vi "rmx13_rev2.vi"() -> ()   [LabVIEW 2012]
uses:
  <vilib>/Utility/inputDevices.llb/closeKeyboard.vi
  <vilib>/Utility/inputDevices.llb/keyboardAcquire.vi
panel:
  in  "Tab Control":enum32{"Front Panel"}(tab)
  out "excavator direction":string="a"
  out "bot direction":string="a"
  out "excavator state":string="a"
  out "hopper state":string="a"
  out "bytes written":i32
  out "tx'd string":string
  out "error out":errorcluster
  in  "Boolean 2":bool
  in  "Boolean":bool
  out "Total Elapsed Time  (HH:MM:SS)":dbl format="%<%H:%M:%S%2u>t"
  out "hup":bool
  out "hdown":bool
  out "xfwd":bool
  out "xback":bool
  out "xdown":bool
  out "xup":bool
  out "right":bool
  out "left":bool
  out "down":bool
  out "up":bool
  # "Excavator State"
  # "Elapsed Time"
  # "Error Control"
  # "Dump Position"
  # "Excavator Direction"
  # "Start/Stop"
  # "Bot Direction"
  # "Hopper State"
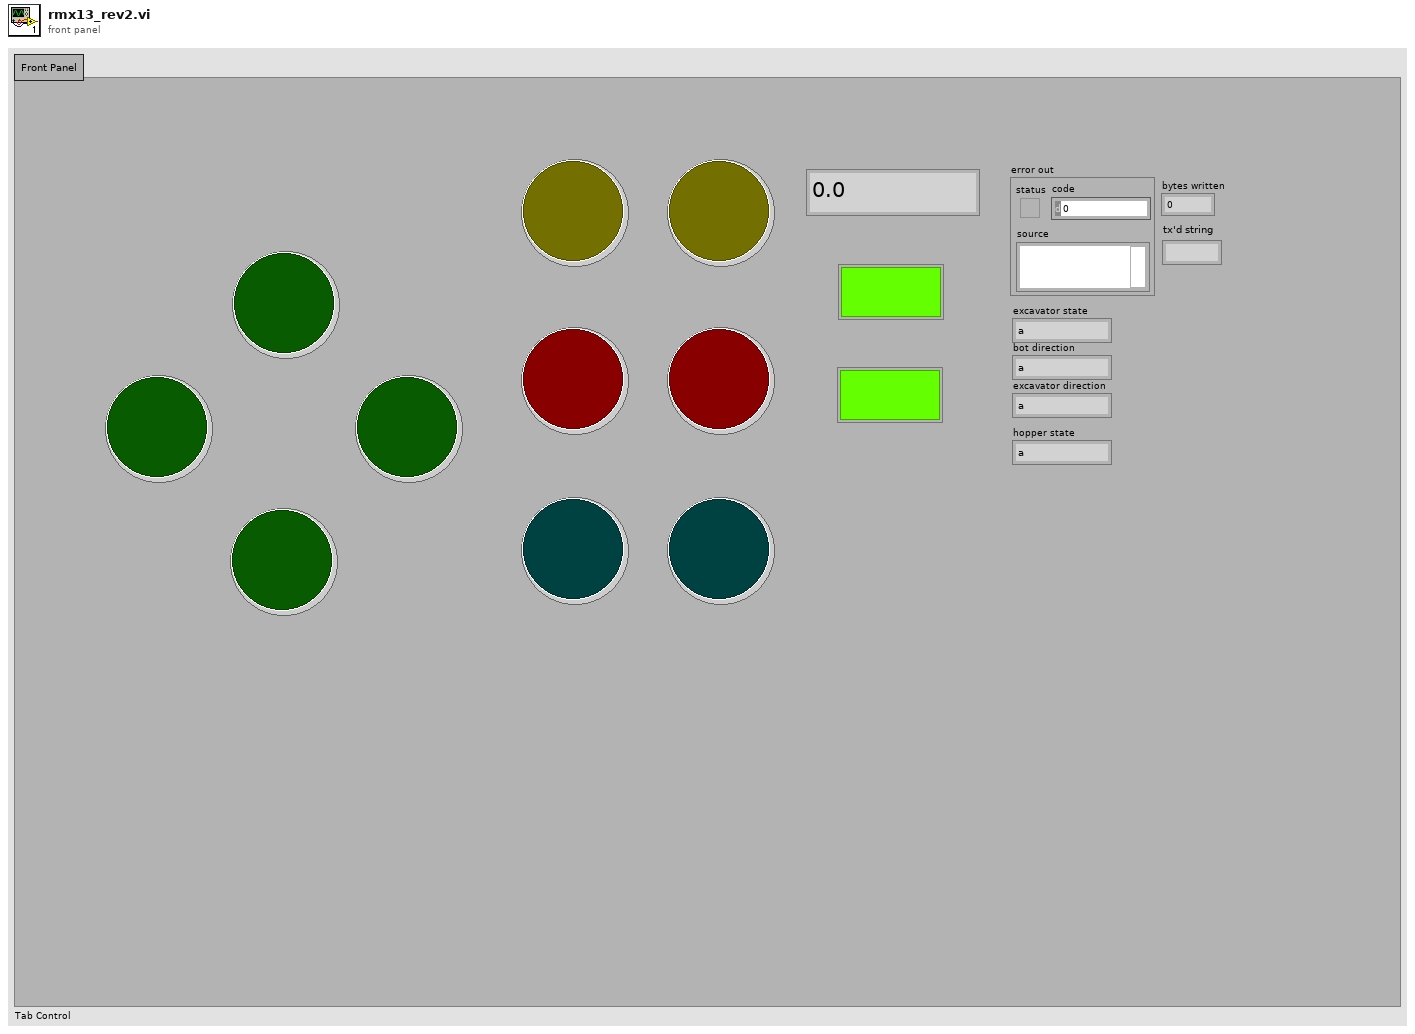
[diagram p1: front panel]
types:
  T1 = enum16{"0", "1", "2", "3", "4", "5", "6", "7", "8", "9", "A", "B", "C", "D", "E", "F", "G", "H", "I", "J", "K", "L", "M", "N", "O", "P", "Q", "R", "S", "T", "U", "V", "W", "X", "Y", "Z", "F1", "F2", "F3", "F4", "F5", "F6", "F7", "F8", "F9", "F10", "F11", "F12", "F13", "F14", "F15", "ADD", "BACK", "BACKSLASH", "CAPITAL", "COMMA", "DECIMAL", "DELETE", "DIVIDE", "DOWN", "END", "EQUALS", "ESCAPE", "GRAVE (`)", "HOME", "INSERT", "LBRACKET", "LCONTROL", "LEFT", "L ALT", "LSHIFT", "LWIN", "MINUS", "MULTIPLY", "NEXT", "NUMLOCK", "NUMPAD_0", "NUMPAD_1", "NUMPAD_2", "NUMPAD_3", "NUMPAD_4", "NUMPAD_5", "NUMPAD_6", "NUMPAD_7", "NUMPAD_8", "NUMPAD_9", "PAUSE", "PERIOD", "PRIOR (PG UP)", "RBRACKET", "RCONTROL", "RETURN", "RIGHT", "R ALT", "RSHIFT", "RWIN", "SCROLL", "SEMICOLON", "SLASH", "SPACE", "SUBTRACT", "TAB", "UP", "ENTER (num pad)", "' (quote)"}[]
  T2 = cluster{"up":bool, "down":bool, "left":bool, "right":bool, "xup":bool, "xdown":bool, "hup":bool, "hdown":bool, "xfwd":bool, "xback":bool}
  T3 = cluster{"bot_dir":string, "x-state":string, "h-state":string, "x-dir":string}
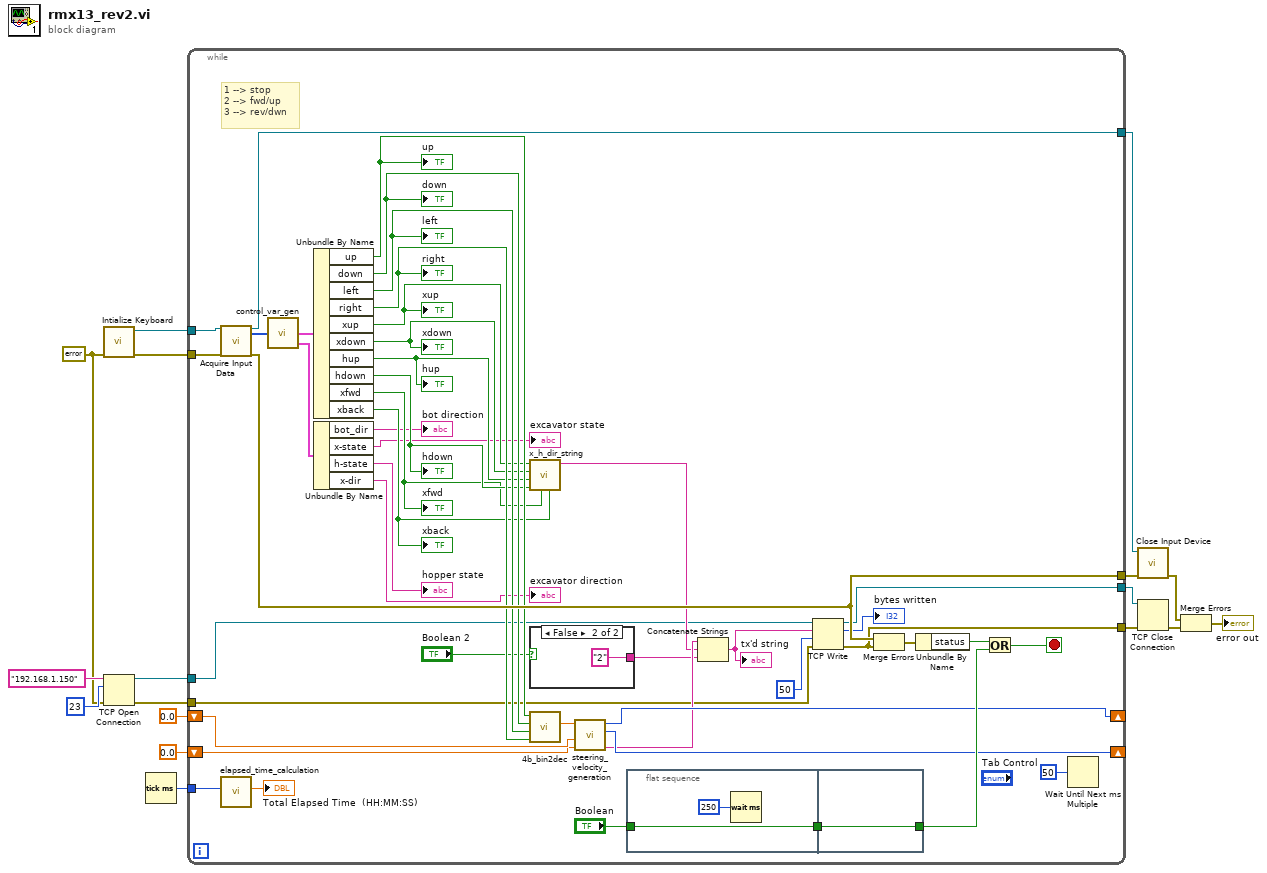
[diagram p0: block diagram]
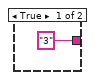
[diagram p2: hidden frame]
diagram:
  w3 = errorcluster {"status"=FALSE, "code"=0, "source"=""} ("error in")
  n1 = call <vilib>:"Intialize Keyboard.vi"("error in (no error)"=w3) -> ("error out"=w16:errorcluster, "device ID"=w17:refnum<k1>)  [unwired: 9 in]
  n2 = TCP Open Connection(address="192.168.1.150", remote port or service name=u16 23, error in (no error)=w3) -> (connection ID=w6:refnum<k5>, error out=w7:errorcluster)  [unwired: 2 in]
  n3 = Tick Count (ms)() -> (millisecond timer value=w13:u32)
  n4 = while {
    tunnel: w17 -> [w63]
    tunnel: w16 -> [w62]
    tunnel: [w59] -> w15
    tunnel: [w51] -> w14
    tunnel: w13 -> [w44]
    shift-right: [w46] -> _
    shift-left: 0.0 -> [w48]
    shift-right: [w45] -> _
    shift-left: 0.0 -> [w47]
    tunnel: w7 -> [w30]
    tunnel: w6 -> [w29]
    tunnel: [w27] -> w5
    tunnel: [w24] -> w4
    stop <- w52 stop-if-true
    # "1 --> stop\n2 --> fwd/up\n3 --> rev/dwn"
    n5 = call-poly <vilib>:"Acquire Input Data.vi"("device ID"=w63, "error in (no error)"=w62) -> ("device ID"=w59:refnum<k1>, "keys pressed"=w58:T1, "error out"=w51:errorcluster)  [unwired: 15 in]
    n6 = call "elapsed_time_calculation.vi"("initial time"=w44) -> ("elapsed time"=→"Total Elapsed Time  (HH:MM:SS)":dbl)  [unwired: 10 in]
    n7 = call "control_var_gen.vi"("keys pressed"=w58) -> ("out_panel"=w57:T2, "out_error"=w56:T3)  [unwired: 5 in]
    n8 = Unbundle By Name(w57) -> ("up"=w42:bool, "down"=w41:bool, "left"=w40:bool, "right"=w39:bool, "xup"=w38:bool, "xdown"=w37:bool, "hup"=w36:bool, "hdown"=w35:bool, "xfwd"=w34:bool, "xback"=w33:bool)
    "up" <- w42
    "down" <- w41
    "left" <- w40
    "right" <- w39
    "xup" <- w38
    "xdown" <- w37
    "hup" <- w36
    "hdown" <- w35
    "xfwd" <- w34
    "xback" <- w33
    n9 = Unbundle By Name(w56) -> ("bot_dir"=→"bot direction":string, "x-state"=→"excavator state":string, "h-state"=→"hopper state":string, "x-dir"=→"excavator direction":string)
    n10 = call "x_h_dir_string.vi"("xback"=w33, "xfwd"=w34, "hdown"=w35, "hup"=w36, "xdown"=w37, "xup"=w38) -> ("x_h_dir"=w31:string)  [unwired: 5 in]
    n11 = case shown="False" "Boolean 2" {
      tunnel: ["3" "2"] -> w25
      frame True {
      }
      frame False {
      }
    }
    n12 = call "4b_bin2dec.vi"("Right"=w39, "Left"=w40, "Down"=w41, "Up"=w42) -> ("Out"=w49:dbl)  [unwired: 7 in]
    n13 = call "steering_velocity_generation.vi"("angular velocity"=w47, "forward velocity"=w48, "bool-to-dec value"=w49) -> ("motor_control_sig"=w32:string, "angular velocity 2"=w45:i32, "forward velocity 2"=w46:i32)  [unwired: 6 in]
    n14 = flat-sequence {
      tunnel: "Boolean" -> [w66]
      tunnel: [w66] -> w61
      tunnel: [w68] -> w53
      tunnel: w61 -> [w68]
      frame #0 {
        n15 = Wait (ms)(milliseconds to wait=u32 250) -> ()  [unwired: 1 out]
      }
      frame #1 {
      }
    }
    n16 = Concatenate Strings(w32, w31, w25) -> (w18:string)
    "tx'd string" <- w18
    n17 = TCP Write(connection ID=w29, data in=w18, error in (no error)=w30, 9:50 ("timeout ms (25000)")) -> (connection ID out=w27:refnum<k5>, bytes written=→"bytes written":i32, error out=w24:errorcluster)
    n18 = Merge Errors(w51, w24) -> (w50:errorcluster)
    n19 = Unbundle By Name(w50) -> ("status"=w54:bool)
    n20 = Or(x=w54, y=w53) -> (x .or. y?=w52:bool)
    n21 = Wait Until Next ms Multiple(millisecond multiple=u32 50) -> ()  [unwired: 1 out]
  }
  n22 = call-poly <vilib>:"Close Input Device.vi"("error in (no error)"=w14, "device ID"=w15) -> ("error out"=w12:errorcluster)  [unwired: 8 in]
  n23 = TCP Close Connection(connection ID=w5, error in (no error)=w4) -> (error out=w2:errorcluster)  [unwired: 1 in, 1 out]
  n24 = Merge Errors(w12, w2) -> (→"error out":errorcluster)
